vi "CL_control.vi"(6 "ResetPID":bool, 8 "Motor_index":i32[](array[numeric])=[3, 6, 9, 12, 2, 7, 8, 13, 4, 5, 10, 11, 1, 14], 9 "sampling freq [Hz]":dbl=1000.0, 10 "curr_Tensions":dbl[](array[numeric]), 11 "goal_Tensions":dbl[](array[numeric])) -> (3 "can_Current":dbl[](array[numeric]), 4 "Reset PID (output)":bool)   [LabVIEW 2024]
uses:
  <vilib>/addons/control/pid/pid.llb/PID Structure.ctl
  <vilib>/addons/control/pid/pid.llb/PID Gain Unit.ctl
  <vilib>/addons/control/pid/pid.llb/PID Time Unit.ctl
  <vilib>/addons/control/pid/pid.llb/PID Structure Conversion (DBL Array).vi
  <vilib>/addons/control/pid/pid.llb/PID (DBL Array).vi
  <vilib>/addons/control/pid/NI_PID_pid.lvlib
panel:
  in  "max/min ctrl effort":cluster{"output high":dbl, "output low":dbl}={"output high"=9577.89, "output low"=-9577.89}
  in  "PID Gains [Parallel]":cluster{"Kp":dbl, "Ki":dbl, "Kd":dbl}[](array[cluster])=[{"Kp"=0.0, "Ki"=0.0, "Kd"=0.0}, {"Kp"=6.0, "Ki"=0.0, "Kd"=0.7}, {"Kp"=6.0, "Ki"=0.0, "Kd"=0.7}, {"Kp"=6.0, "Ki"=0.0, "Kd"=0.7}, {"Kp"=6.0, "Ki"=0.0, "Kd"=0.7}, {"Kp"=6.0, "Ki"=0.0, "Kd"=0.7}, {"Kp"=6.0, "Ki"=0.0, "Kd"=0.7}, {"Kp"=6.0, "Ki"=0.0, "Kd"=0.7}, {"Kp"=6.0, "Ki"=0.0, "Kd"=0.7}, {"Kp"=6.0, "Ki"=0.0, "Kd"=0.7}, {"Kp"=6.0, "Ki"=0.0, "Kd"=0.7}, {"Kp"=6.0, "Ki"=0.0, "Kd"=0.7}, {"Kp"=6.0, "Ki"=0.0, "Kd"=0.7}, {"Kp"=0.0, "Ki"=0.0, "Kd"=0.0}]
  # "66.1 Amp Stall Current\n\nmax achievable instantaneous\nTension Command\n\n66100 * 0.1449 = 9577.89 N"
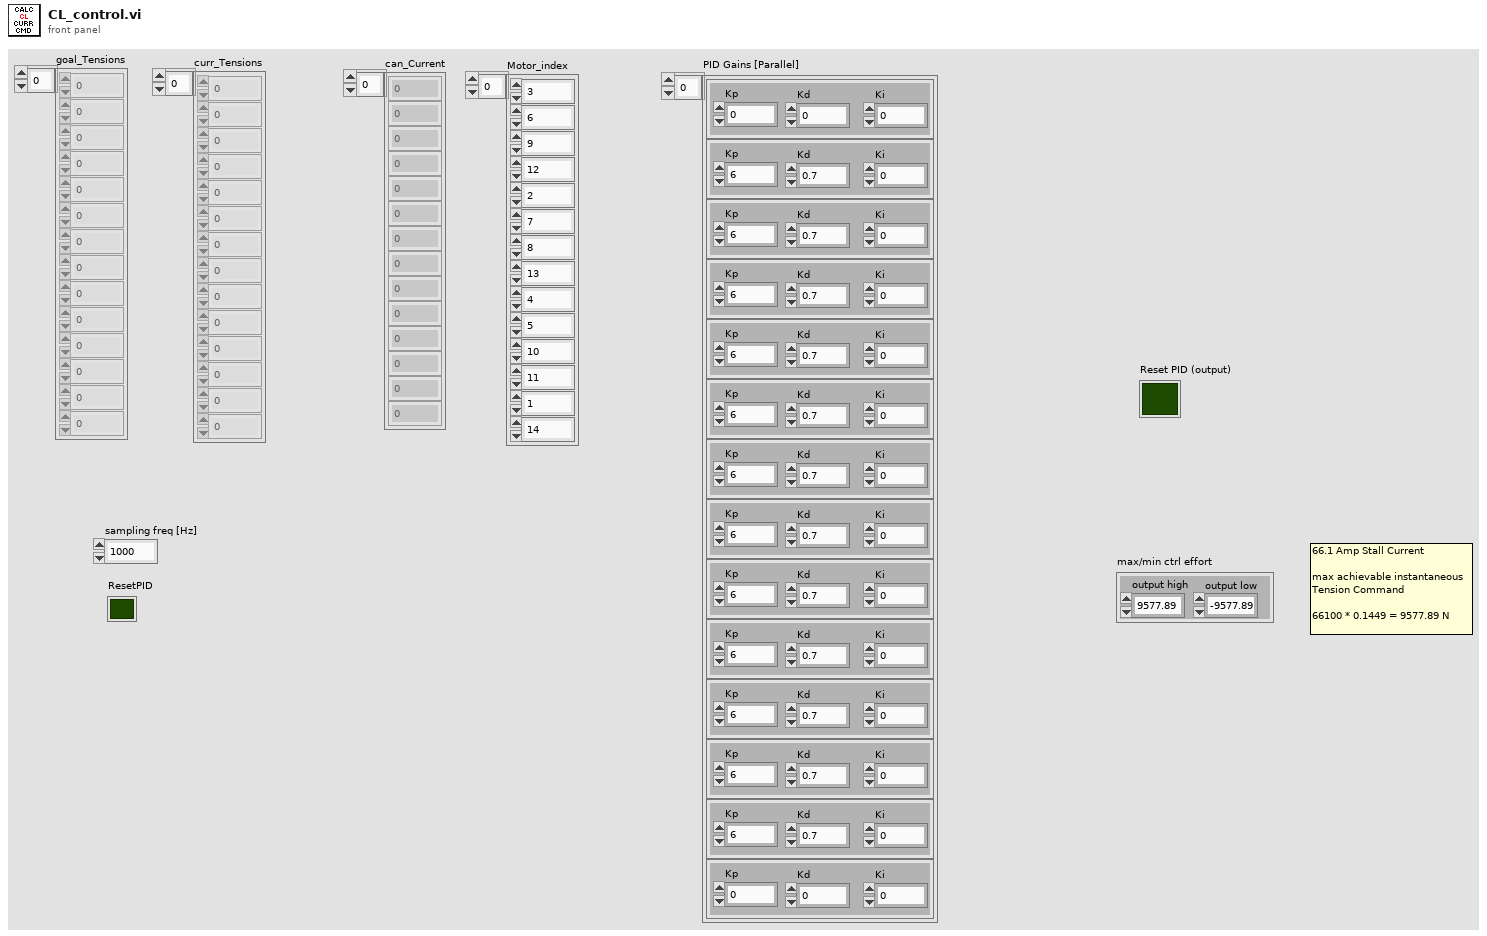
[diagram p1: front panel]
types:
  T1 = typedef "NI_PID_pid.lvlib/PID Time Unit.ctl" = u16
  T2 = typedef "NI_PID_pid.lvlib/PID Gain Unit.ctl" = u16
  T3 = typedef "NI_PID_pid.lvlib/PID Structure.ctl" = u16
  T4 = cluster{"proportional gain (Kc)":dbl, "integral time (Ti, min)":dbl, "derivative time (Td, min)":dbl}[]
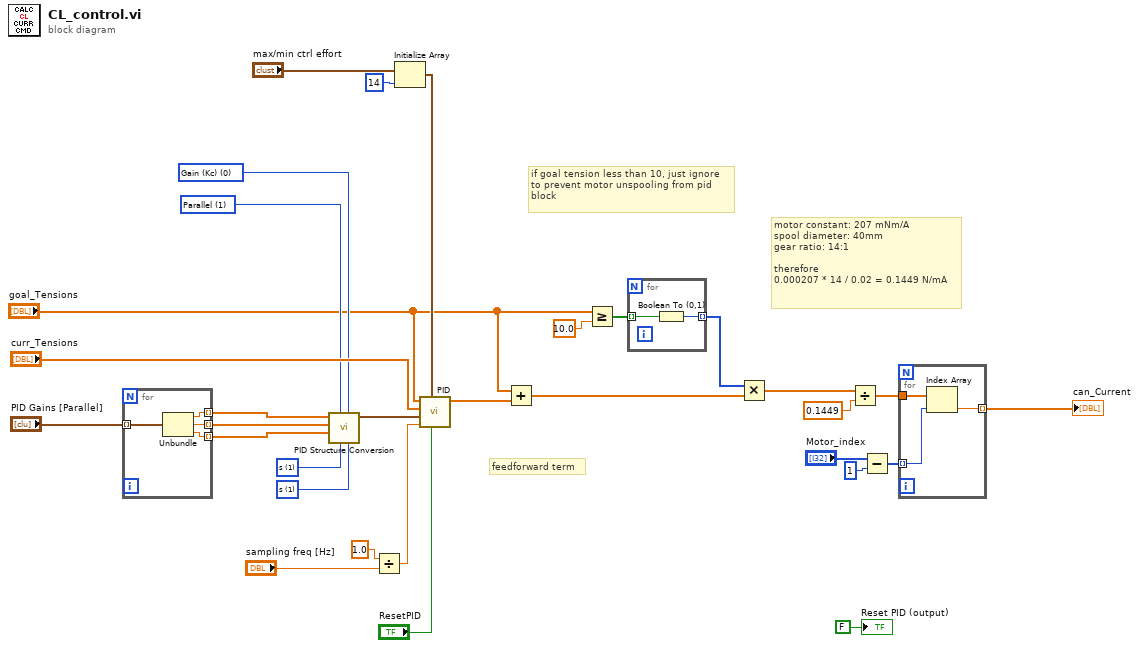
[diagram p0: block diagram]
diagram:
  w18 = T1 1 items=["min", "s"] ("derivative unit")
  w19 = T1 1 items=["min", "s"] ("integral unit")
  w20 = T2 0 items=["Gain (Kc)", "Band (PB)"] ("proportional unit")
  w21 = T3 1 items=["Academic (Standard)", "Parallel", "Series"] ("PID structure")
  # "feedforward term"
  # "if goal tension less than 10, just ignore\nto prevent motor unspooling from pid\nblock"
  # "motor constant: 207 mNm/A\nspool diameter: 40mm\ngear ratio: 14:1\n\ntherefore\n0.000207 * 14 / 0.02 = 0.1449 N/mA"
  n1 = for {
    tunnel: "PID Gains [Parallel]" -> [w35] mode=indexing
    tunnel: [w34] -> w14 mode=indexing
    tunnel: [w33] -> w16 mode=indexing
    tunnel: [w32] -> w15 mode=indexing
    n2 = Unbundle(w35) -> ("Kp"=w32:dbl, "Ki"=w33:dbl, "Kd"=w34:dbl)
  }
  n3 = call-poly <vilib>:"PID Structure Conversion.vi"("derivative unit"=w18, "proportional unit"=w20, "integral unit"=w19, "PID structure"=w21, "derivative"=w14, "integral"=w16, "proportional"=w15) -> ("PID parameters"=w13:T4)  [unwired: 4 in]
  n4 = Divide(x=1.0, y="sampling freq [Hz]") -> (x/y=w29:dbl)
  n5 = Initialize Array("max/min ctrl effort", 14 ("dimension size")) -> (w4:cluster{"output high":dbl, "output low":dbl}[])
  n6 = call-poly <vilib>:"PID.vi"("reinitialize? (F)"="ResetPID", "output range"=w4, "dt (s)"=w29, "PID gains"=w13, "process variable"="curr_Tensions", "setpoint"="goal_Tensions") -> ("output"=w2:dbl[])  [unwired: 4 in, 1 out]
  n7 = Add(x="goal_Tensions", y=w2) -> (x+y=w3:dbl[])
  n8 = Greater Or Equal?(x="goal_Tensions", y=10.0) -> (x >= y?=w8:bool[])
  n9 = for {
    tunnel: w8 -> [w37] mode=indexing
    tunnel: [w36] -> w7 mode=indexing
    n10 = Boolean To (0,1)(Boolean=w37) -> (0, 1=w36:i16)
  }
  n11 = Multiply(x=w7, y=w3) -> (x*y=w9:dbl[])
  n12 = Divide(x=w9, y=0.1449) -> (x/y=w23:dbl[])
  n13 = Subtract(x="Motor_index", y=1) -> (x-y=w25:i32[])
  n14 = for {
    tunnel: w25 -> [w40] mode=indexing
    tunnel: w23 -> [w39]
    tunnel: [w38] -> w28 mode=indexing
    n15 = Index Array(array=w39, index=w40) -> (element=w38:dbl)
  }
  "can_Current" <- w28
  "Reset PID (output)" <- FALSE
